vi "Periodic Tasks.vi"(8 "error in":errorcluster) -> ()   [LabVIEW 2017]
doc: "This VI runs in parallel to other tasks. It can contain as many user-defined periodic loops as you need. These can carry out PID or other sorts of timed response."
uses:
  <vilib>/Rock Robotics/WPI/Utilities/WPI_GetSetVariantRefNum.vi
  <vilib>/Rock Robotics/WPI/ThirdParty/Phoenix-LabVIEW/Pigeon IMU/CTRE_PigeonIMU_GetYPR.vi
  <vilib>/Rock Robotics/Network Tables/NT Write Number.vi
  <vilib>/Rock Robotics/SystemInterfaces/AI/FPGA_AIChannel.ctl
  <vilib>/Rock Robotics/WPI/Ultrasonic/WPI_SonarMB1010AnalogGetRange.vi
  <vilib>/Rock Robotics/WPI/Ultrasonic/WPI_SonarMB1010AnalogClose.vi
  <vilib>/Rock Robotics/WPI/Ultrasonic/WPI_SonarMB1010AnalogOpen.vi
  <vilib>/Rock Robotics/WPI/Ultrasonic/WPI_SonarMB1010AnalogRefNum Registry Set.vi
panel:
  out "Yaw Pitch Roll 2":cluster{"Yaw":dbl, "Pitch":dbl, "Roll":dbl}
  out "Yaw Pitch Roll":cluster{"Yaw":dbl, "Pitch":dbl, "Roll":dbl}
  out "distance":dbl(slide)=125.0 scale=0.0..250.0 scale format="%3d"
  in  "Scaling Factor":dbl=0.025
  in  "Average Bits":u8=3 max=15
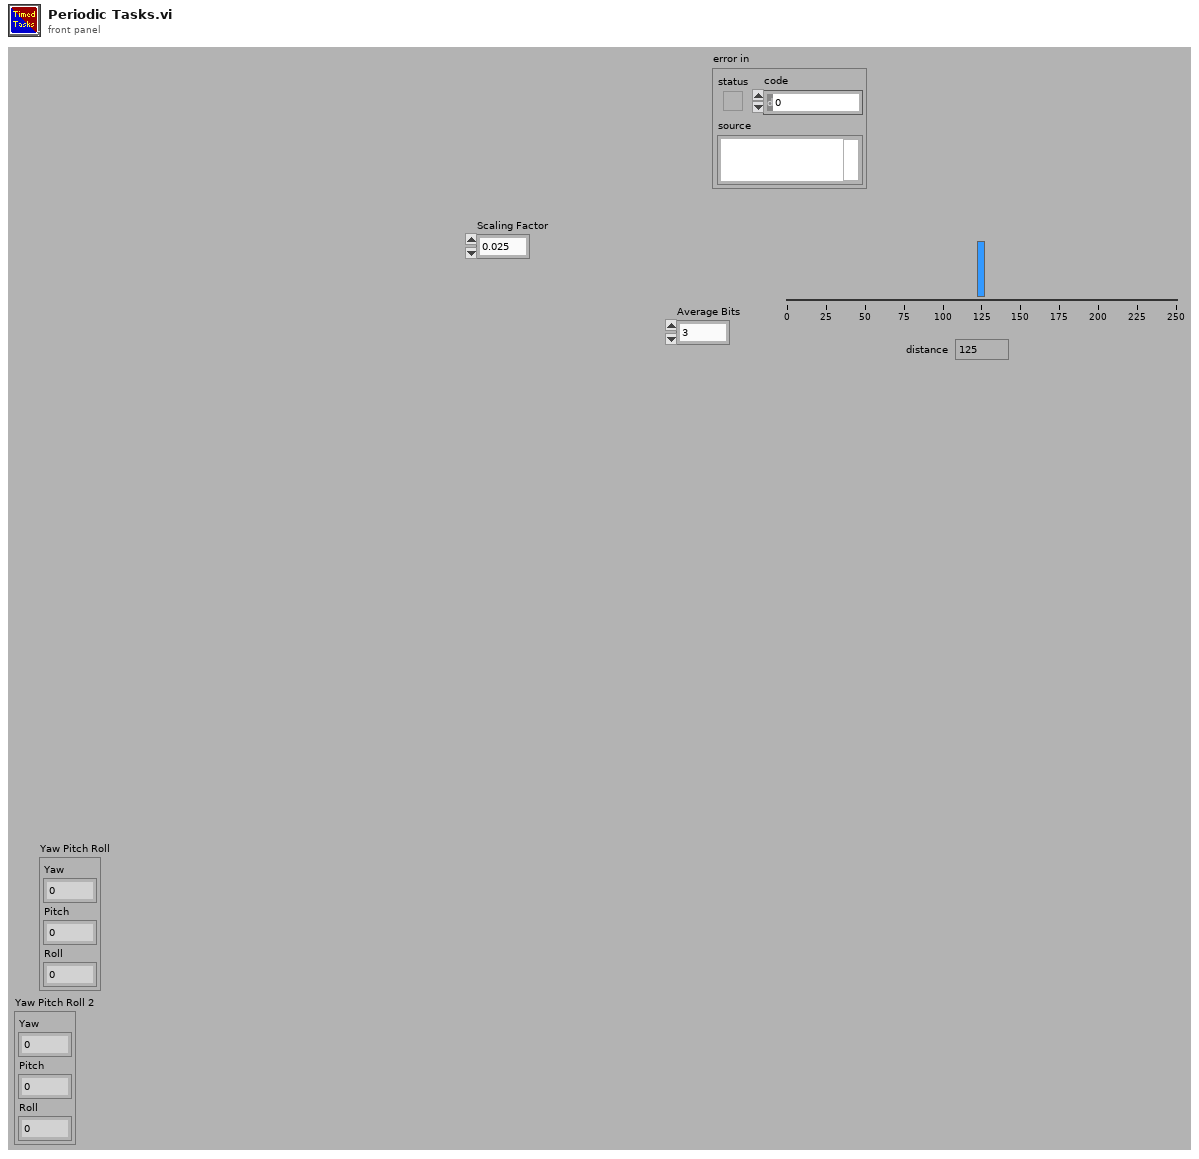
[diagram p1: front panel]
types:
  T1 = typedef "CTRE_PigeonIMU_DeviceRef.ctl" = cluster{"DeviceStatus":errorcluster, "Device Number":u8, "Type":T2, "Device ID":u32, "Handle":u64, "UsageFrame":u32, "Library Path":path}
  T2 = typedef "CTRE_PigeonIMU_ConnectionType.ctl" = u32
  T3 = typedef "FPGA_AIChannel.ctl" = enum8{"AI 0", "AI 1", "AI 2", "AI 3", "AI MXP 0", "AI MXP 1", "AI MXP 2", "AI MXP 3", "Invalid"}
  T4 = typedef "WPI_SonarMB1010AnalogDeviceRef.ctl" = cluster{"AIDeviceRef":T5, "Scaling factor (V/in)":dbl, "Average Bits":u8}
  T5 = typedef "WPI_AnalogChannelDevRef.ctl" = cluster{"DevStatus":errorcluster, "Analog Channel":T3}
  T6 = typedef "WPI_RobotDriveDevRef.ctl" = cluster{"DevStatus":errorcluster, "Motors[]":T7[], "Square Inputs":bool, "Max Output":dbl}
  T7 = typedef "WPI_MotorControlDeviceRef.ctl" = cluster{"DeviceStatus":errorcluster, "Type":T8, "PWM":cluster{"PWM Channel":T9, "DeadBand":T10}, "CAN":cluster{"Device Number":u8, "SetOutput VI Ref":variant, "GetOutput VI Ref":variant, "Enable VI Ref":variant, "Disable VI Ref":variant, "Data":variant}, "Invert":bool, "DIO PWM":cluster{"PWM \"Enable\" Channel":T9, "DIOChannel":T11, "PWM Rate":dbl}}
  T8 = typedef "WPI_MotorControlType.ctl" = enum16{"PWM", "CAN", "DIO PWM"}
  T9 = typedef "FPGA_DIOPWMChannel.ctl" = enum8{"PWM 0", "PWM 1", "PWM 2", "PWM 3", "PWM 4", "PWM 5", "PWM 6", "PWM 7", "PWM 8", "PWM 9", "PWM MXP 0", "PWM MXP 1", "PWM MXP 2", "PWM MXP 3", "PWM MXP 4", "PWM MXP 5", "PWM MXP 6", "PWM MXP 7", "PWM MXP 8", "PWM MXP 9", "Invalid"}
  T10 = typedef "WPI_PWMDeadband.ctl" = cluster{"Name":string, "maxPositivePwm":i32, "minPositivePwm":i32, "centerPwm":i32, "maxNegativePwm":i32, "minNegativePwm":i32, "angularRange":u16}
  T11 = typedef "FPGA_DIOChannel.ctl" = enum8{"DIO 0", "DIO 1", "DIO 2", "DIO 3", "DIO 4", "DIO 5", "DIO 6", "DIO 7", "DIO 8", "DIO 9", "DIO MXP 0", "DIO MXP 1", "DIO MXP 2", "DIO MXP 3", "DIO MXP 4", "DIO MXP 5", "DIO MXP 6", "DIO MXP 7", "DIO MXP 8", "DIO MXP 9", "DIO MXP 10", "DIO MXP 11", "DIO MXP 12", "DIO MXP 13", "DIO MXP 14", "DIO MXP 15", "SPI Port CS1", "SPI Port CS2", "SPI Port CS3", "SPI Port MISO", "SPI Port MOSI", "Invalid"}
  T12 = typedef "WPI_JoystickDevRef.ctl" = cluster{"Device":T13}
  T13 = typedef "WPI_JoystickDeviceEnum.ctl" = enum16{"USB 0", "USB 1", "USB 2", "USB 3", "USB 4", "USB 5"}
  T14 = cluster{"JoystickDevRef":T12, "RobotDriveDevRef":T6}
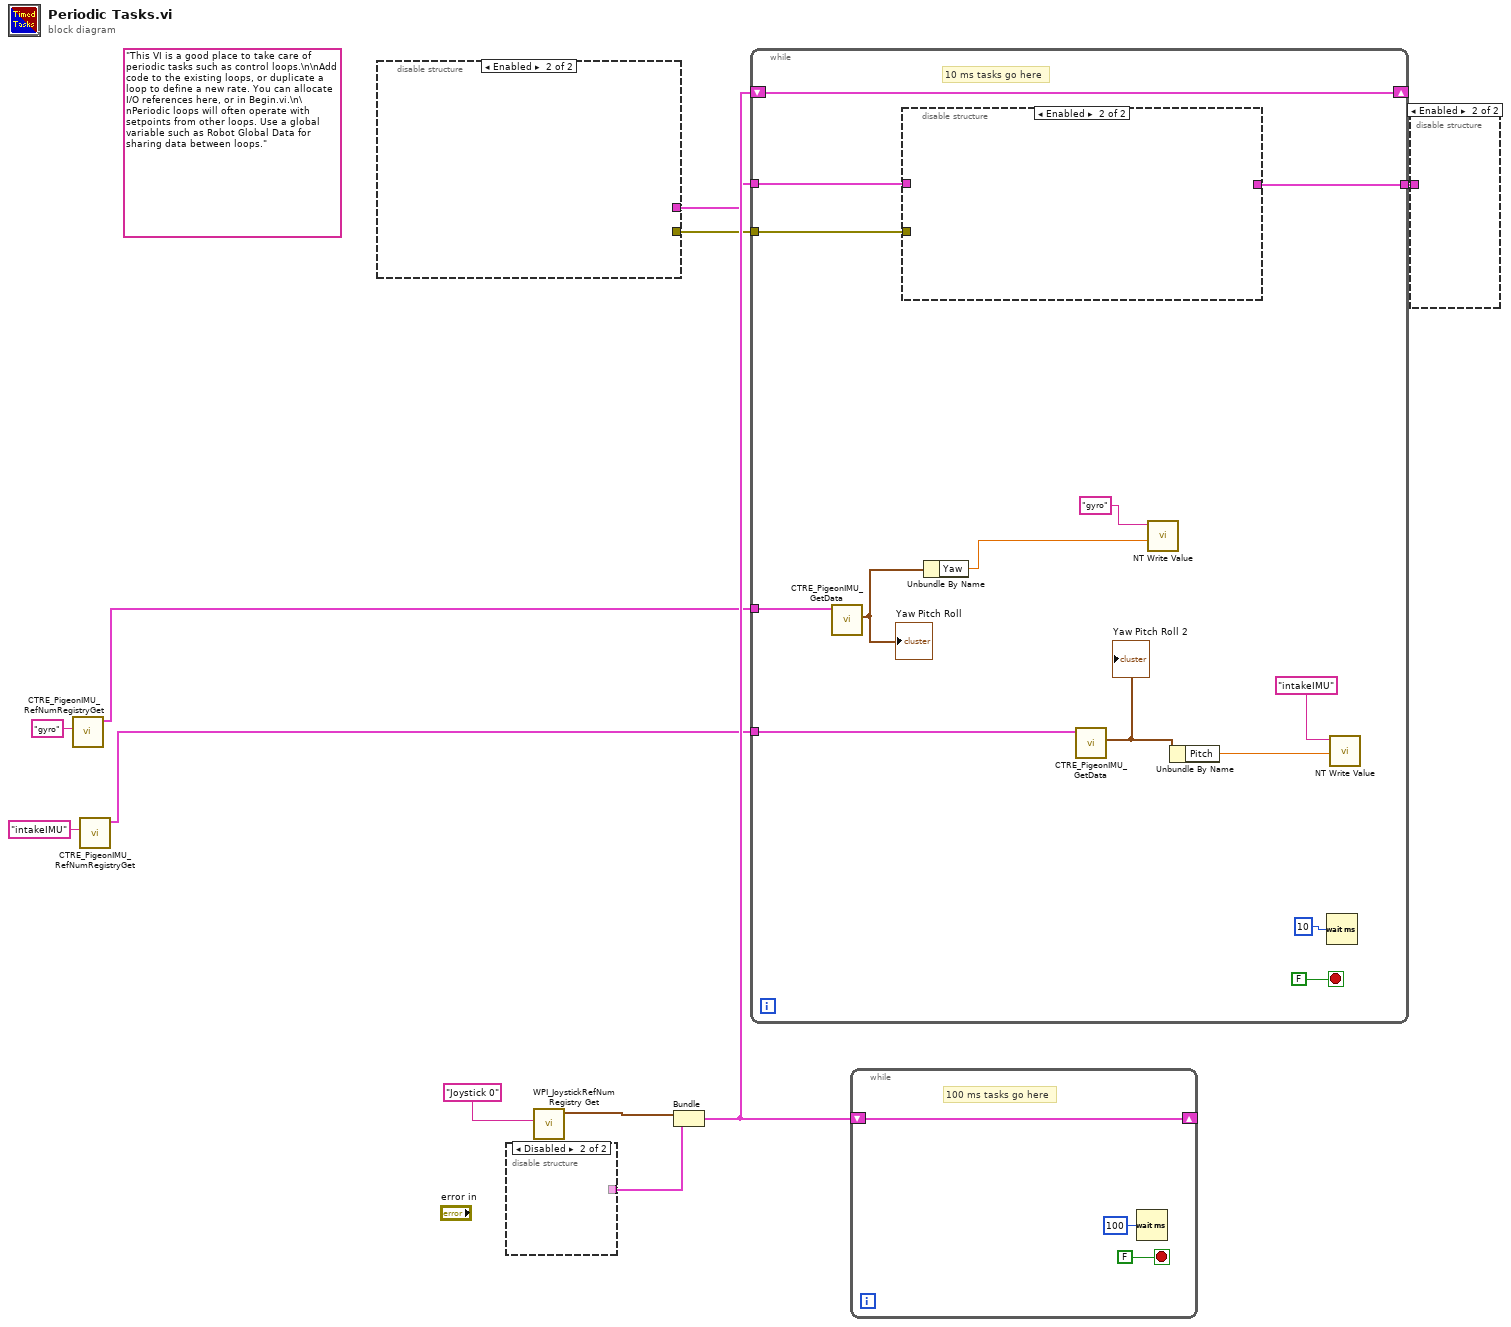
[diagram p0: block diagram]
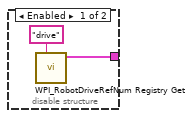
[diagram p2: hidden frame]
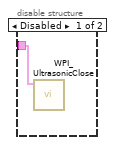
[diagram p3: hidden frame]
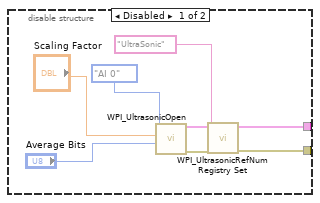
[diagram p4: hidden frame]
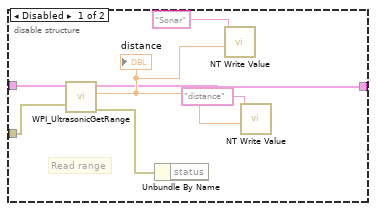
[diagram p5: hidden frame]
diagram:
  (unwired) "This VI is a good place to take care of periodic tasks such as control loops.\n\nAdd code to the existing loops, or duplicate a loop to define a new rate. You can allocate I/O references here, or in Begin.vi.\n\nPeriodic loops will often operate with setpoints from other loops. Use a global variable such as Robot Global Data for sharing data between loops."
  n1 = call <vilib>:"CTRE_PigeonIMU_RefNumRegistryGet.vi"("refnum name"="gyro") -> ("PigeonIMUDevRef"=w1:T1)  [unwired: 9 in, 1 out]
  n2 = call <vilib>:"CTRE_PigeonIMU_RefNumRegistryGet.vi"("refnum name"="intakeIMU") -> ("PigeonIMUDevRef"=w2:T1)  [unwired: 9 in, 1 out]
  n3 = disable-structure shown="Enabled" {
    disable-tunnel: [w13 _] -> w7
    disable-tunnel: [w12 _] -> w6
    frame Disabled {
      n4 = call-poly <vilib>:"WPI_UltrasonicOpen.vi"("Average Bits"="Average Bits", "Scaling factor (V/in)"="Scaling Factor", "Analog Channel"=FPGA_AIChannel."AI 0") -> ("error out"=w17:errorcluster, "SonarMB1010AnalogDevRef"=w15:T4)  [unwired: 7 in]
      n5 = call-poly <vilib>:"WPI_UltrasonicRefNum Registry Set.vi"("error in (no error)"=w17, "refnum name"="UltraSonic", "SonarMB1010AnalogDevRef"=w15) -> ("error out"=w12:errorcluster, "SonarMB1010AnalogDevRef"=w13:T4)  [unwired: 7 in]
    }
    frame Enabled {
    }
  }
  n6 = disable-structure shown="Disabled" {
    disable-tunnel: [w20 _] -> w9
    frame Enabled {
      n7 = call <vilib>:"WPI_RobotDriveRefNum Registry Get.vi"("refnum name"="drive") -> ("RobotDriveDevRef"=w20:T6)  [unwired: 1 in, 9 out]
    }
    frame Disabled {
    }
  }
  n8 = call <vilib>:"WPI_JoystickRefNum Registry Get.vi"("refnum name"="Joystick 0") -> ("JoystickDevRef"=w10:T12)  [unwired: 1 in, 9 out]
  n9 = Bundle("JoystickDevRef"=w10, "RobotDriveDevRef"=w9) -> (w8:T14)  [unwired: 1 out]
  n10 = while {
    shift-right: [w33] -> _
    shift-left: w8 -> [w33]
    tunnel: w7 -> [w32]
    tunnel: w6 -> [w31]
    tunnel: [w30] -> w5
    tunnel: w2 -> [w24]
    tunnel: w1 -> [w23]
    stop <- FALSE stop-if-true
    # "10 ms tasks go here"
    n11 = call-poly <vilib>:"CTRE_PigeonIMU_GetData.vi"("PigeonIMUDevRef"=w23) -> ("Yaw Pitch Roll"=w26:cluster{"Yaw":dbl, "Pitch":dbl, "Roll":dbl})  [unwired: 8 in, 2 out]
    "Yaw Pitch Roll" <- w26
    n12 = disable-structure shown="Enabled" {
      disable-tunnel: w32 -> [w38 _]
      disable-tunnel: w31 -> [w37 _]
      disable-tunnel: [w36 _] -> w30
      frame Disabled {
        # "Read range"
        n13 = call-poly <vilib>:"WPI_UltrasonicGetRange.vi"("error in"=w37, "SonarMB1010AnalogDevRef"=w38) -> ("error out"=w42:errorcluster, "Distance"=w40:dbl, "SonarMB1010AnalogDevRef"=w36:T4)  [unwired: 7 in]
        "distance" <- w40
        n14 = Unbundle By Name(w42) -> ()  [unwired: 1 out]
        n15 = call-poly <vilib>:"NT Write Value.vi"("Numeric"=w40, "Name"="Sonar") -> ()  [unwired: 9 in, 1 out]
        n16 = call-poly <vilib>:"NT Write Value.vi"("Numeric"=w40, "Name"="distance") -> ()  [unwired: 9 in, 1 out]
      }
      frame Enabled {
      }
    }
    n17 = Unbundle By Name(w26) -> ("Yaw"=w27:dbl)
    n18 = call-poly <vilib>:"CTRE_PigeonIMU_GetData.vi"("PigeonIMUDevRef"=w24) -> ("Yaw Pitch Roll"=w28:cluster{"Yaw":dbl, "Pitch":dbl, "Roll":dbl})  [unwired: 8 in, 2 out]
    "Yaw Pitch Roll 2" <- w28
    n19 = call-poly <vilib>:"NT Write Value.vi"("Numeric"=w27, "Name"="gyro") -> ()  [unwired: 9 in, 1 out]
    n20 = Unbundle By Name(w28) -> ("Pitch"=w29:dbl)
    n21 = Wait (ms)(milliseconds to wait=u32 10) -> ()  [unwired: 1 out]
    n22 = call-poly <vilib>:"NT Write Value.vi"("Numeric"=w29, "Name"="intakeIMU") -> ()  [unwired: 9 in, 1 out]
  }
  n23 = while {
    shift-right: [w43] -> _
    shift-left: w8 -> [w43]
    stop <- FALSE stop-if-true
    # "100 ms tasks go here"
    n24 = Wait (ms)(milliseconds to wait=u32 100) -> ()  [unwired: 1 out]
  }
  n25 = disable-structure shown="Enabled" {
    disable-tunnel: w5 -> [w46 _]
    frame Disabled {
      n26 = call-poly <vilib>:"WPI_UltrasonicClose.vi"("SonarMB1010AnalogDevRef"=w46) -> ()  [unwired: 10 in, 1 out]
    }
    frame Enabled {
    }
  }
